vi "SetWidthAndHeightInXLS.vi"() -> ()   [LabVIEW 2014]
uses:
  Typedefs/Worksheet Format.ctl
  C:/PhaeronGit/LVNPOI/Resources/NPOI 2.1.1 dotnet2/NPOI.dll
  Resources/NPOI 2.1.1 dotnet2/NPOI.dll
panel:
  in  "Worksheet Format (XLSX)":T1
  in  "sheetname":string="Sheet1"
  in  "File Name":path=path "C:/PhaeronGit/LVNPOI/Scratch/test.xlsx"
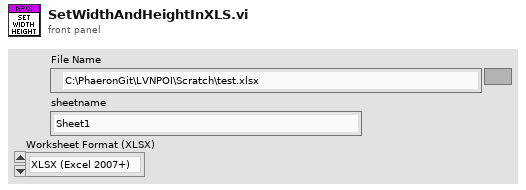
[diagram p1: front panel]
types:
  T1 = typedef "Worksheet Format.ctl" = enum16{"XLSX (Excel 2007+)", "XLS (Excel Legacy)"}
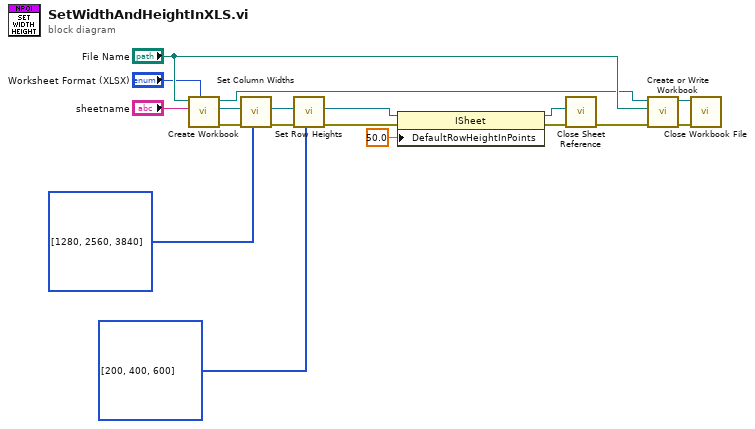
[diagram p0: block diagram]
diagram:
  n1 = call "Create Workbook.vi"("Worksheet Format (XLSX)"="Worksheet Format (XLSX)", "Sheetname (Sheet1)"="sheetname", "File Name"="File Name") -> ("error out"=w2:errorcluster, "Sheet Reference"=w3:refnum<k24>, "IWorkbook Reference"=w4:refnum<k24>)  [unwired: 6 in]
  n2 = call "Set Column Widths.vi"("Column Widths"=i32[] [1280, 2560, 3840], "error in (no error)"=w2, "Sheet Reference"=w3) -> ("error out"=w15:errorcluster, "Sheet Reference out"=w16:refnum<k24>)  [unwired: 7 in]
  n3 = call "Set Row Heights.vi"("Row Heights"=i16[] [200, 400, 600], "error in (no error)"=w15, "Sheet Reference"=w16) -> ("error out"=w12:errorcluster, "Sheet Reference out"=w13:refnum<k24>)  [unwired: 7 in]
  n4 = property class="ISheet"(reference=w13, error in=w12, "DefaultRowHeightInPoints"=sgl 50.0) -> (reference out=w10:refnum<k24>, error out=w11:errorcluster)
  n5 = call "Close Sheet Reference.vi"("error in (no error)"=w11, "Sheet Reference"=w10) -> ("error out"=w9:errorcluster)  [unwired: 9 in]
  n6 = call "Create or Write Workbook.vi"("error in (no error)"=w9, "File Name"="File Name", "IWorkbook Reference"=w4) -> ("error out"=w8:errorcluster, "IWorkbook Reference Out"=w7:refnum<k24>)  [unwired: 7 in]
  n7 = call "Close Workbook File.vi"("error in (no error)"=w8, "IWorkbook Reference"=w7) -> ()  [unwired: 9 in, 1 out]
